vi "PPMS_Repeticiones.vi"() -> (0 "Ciclos":i32, 3 "Cancelled?":bool)   [LabVIEW 2017]
doc: "Use this template to create a dialog box. This template polls the state of the buttons on the front panel and does not use events. Use the Dialog Using Events template (not available in Base package) to create a dialog box with event handling."
panel:
  in  "Ciclos":i32=10
  in  "Cancel":bool
  in  "OK":bool
  # "Número de repeticiones"
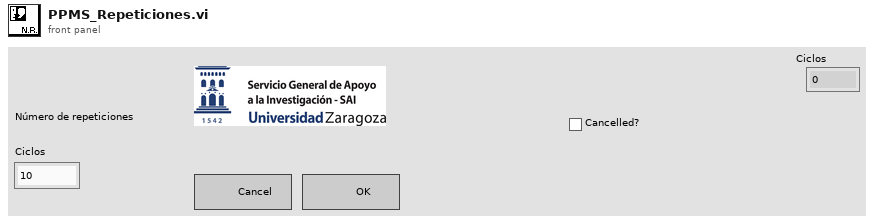
[diagram p1: front panel]
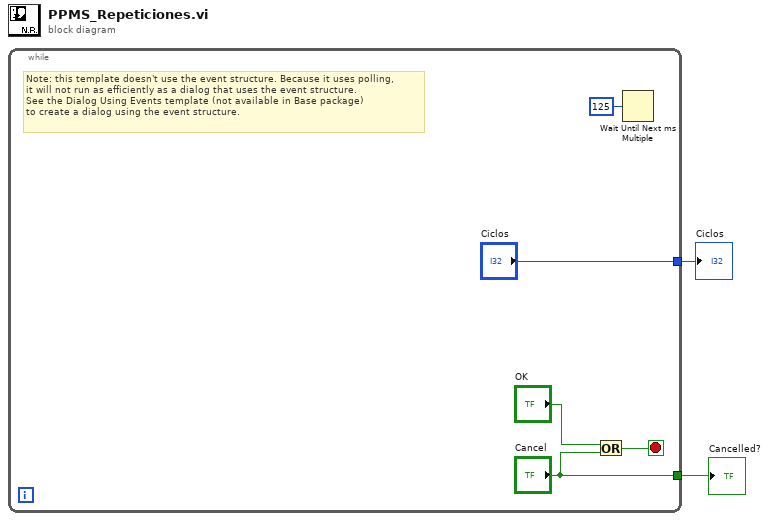
[diagram p0: block diagram]
diagram:
  n1 = while {
    tunnel: ["Cancel"] -> w2
    tunnel: ["Ciclos"] -> w1
    stop <- w6 stop-if-true
    # "Note: this template doesn't use the event structure. Because it uses polling, \nit will not run as efficiently as a dialog that uses the event structure.\nSee the Dialog Using Events template (not available in Base package) \nto create a dialog using the event structure."
    n2 = Or(x="OK", y="Cancel") -> (x .or. y?=w6:bool)
    n3 = Wait Until Next ms Multiple(millisecond multiple=u32 125) -> ()  [unwired: 1 out]
  }
  "Cancelled?" <- w2
  "Ciclos" <- w1
